vi "Set DA Cm V.vi"(8 "error in (no error)":errorcluster, 10 "vol_mv":i32, 11 "channel":u8) -> (0 "error out":errorcluster)   [LabVIEW 2021, in "vmmso.lvlib"]
doc: "DLL_API void WINAPI SetDACmV(unsigned char channel, int vol_mv);"
uses:
  vmmso.lvlib
  vmmso.dll
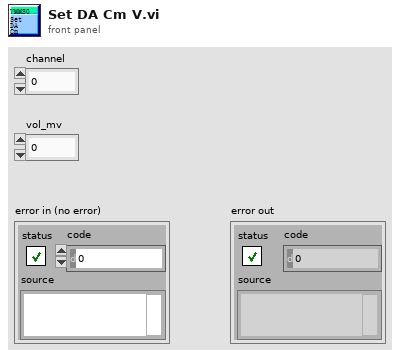
[diagram p1: front panel]
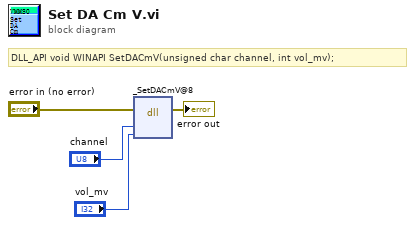
[diagram p0: block diagram]
diagram:
  # "DLL_API void WINAPI SetDACmV(unsigned char channel, int vol_mv);"
  n1 = dll-call lib="O:/MSO/library/demo-Labview/vmmso/vmmso.*" fn="_SetDACmV@8"(error in="error in (no error)", "channel"="channel", "vol_mv"="vol_mv") -> (error out=→"error out":errorcluster)  [unwired: 5 in, 1 out]
